vi "Disconnect.vi"(8 "error in (no error)":errorcluster, 11 "HamaCam in":refnum<class "HamaCam.lvclass">) -> (0 "error out":errorcluster, 3 "HamaCam out":refnum<class "HamaCam.lvclass">)   [LabVIEW 2023, in "HamaCam.lvlib" / "HamaCam.lvclass"]
uses:
  HamaCam.lvclass
  HamaCam.lvclass/HamaCam.ctl
  <vilib>/ActorFramework/Actor/Actor.lvclass
  Interfaces/InitDeinitInterface/InitDeinitComm Messages/Disconnected Msg/Disconnected Msg.lvclass
  Applications/National Instruments/LabVIEW 2023 64-bit/vi.lib/ActorFramework/Actor/Actor.lvclass
  Users/alexandrosspiliotis/Documents/LV_DAQ_Project/ConcreteClasses/ConcreteInstrumentClasses/CameraClasses/Hama_LV/HamaCam/HamaCam/HamaCam.lvclass
  Users/alexandrosspiliotis/Documents/LV_DAQ_Project/Interfaces/AbstractInstrumentClasses/Cameras_LV/CameraInterface/CameraInterface.lvclass
  Users/alexandrosspiliotis/Documents/LV_DAQ_Project/Interfaces/InitDeinitInterface/InitDeinit/InitDeinit.lvclass
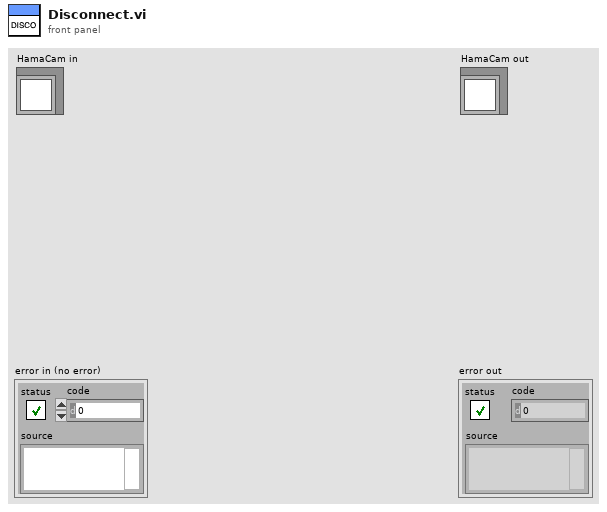
[diagram p1: front panel]
types:
  T1 = typedef "InstrumentData.ctl" = cluster{"Instr Error":errorcluster, "Address":cluster{"address type":enum16{"VISA", "Index"}, "Address":string, "instrument type":T2}}
  T2 = typedef "instrumentType.ctl" = enum16{"Spectrometer", "Camera", "Stepper"}
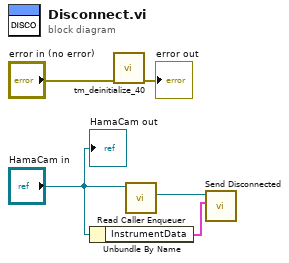
[diagram p0: block diagram]
diagram:
  n1 = Unbundle By Name("HamaCam in") -> ("InstrumentData"=w2:T1)
  n2 = call "tm_deinitialize_40.vi"("error in (no error)"="error in (no error)") -> ("error out"=→"error out":errorcluster)  [unwired: 10 in]
  n3 = call <vilib>:"Read Caller Enqueuer.vi"("Actor"="HamaCam in") -> ("Caller Enqueuer"=w1:refnum<class "Message Enqueuer.lvclass">)  [unwired: 10 in]
  n4 = call "Send Disconnected.vi"("InstrumentData"=w2, "Message Enqueuer"=w1) -> ()  [unwired: 8 in, 2 out]
  "HamaCam out" <- "HamaCam in"
